vi "Video stream.vi"(0 "VideoMode":u32, 1 "Interface name":T1="cam0", 5 "Video codec":string="Microsoft Video 1", 9 "FPS":u32=30, 11 "Video directory path":path=path "C:/test", 12 "Video name":string="test", 13 "Write video":bool, 14 "Quality":i32=750 max=1000) -> (15 "Error Out":errorcluster)   [LabVIEW 2015]
uses:
  <vilib>/userdefined/High Color/IMAQdx.ctl
  <vilib>/vision/driver/IMAQdx.llb/IMAQdx Camera Control Mode.ctl
  <vilib>/vision/Avi.llb/IMAQ AVI2 Refnum.ctl
  <vilib>/vision/driver/NI_Vision_Acquisition_Software.lvlib
  <resource>/objmgr/imaqdx.rc
panel:
  in  "Stop":bool
  out "Video":T2(plugin-control)
  # "PN 27/11/2014, 27/08/2015 (layout change for web window)"
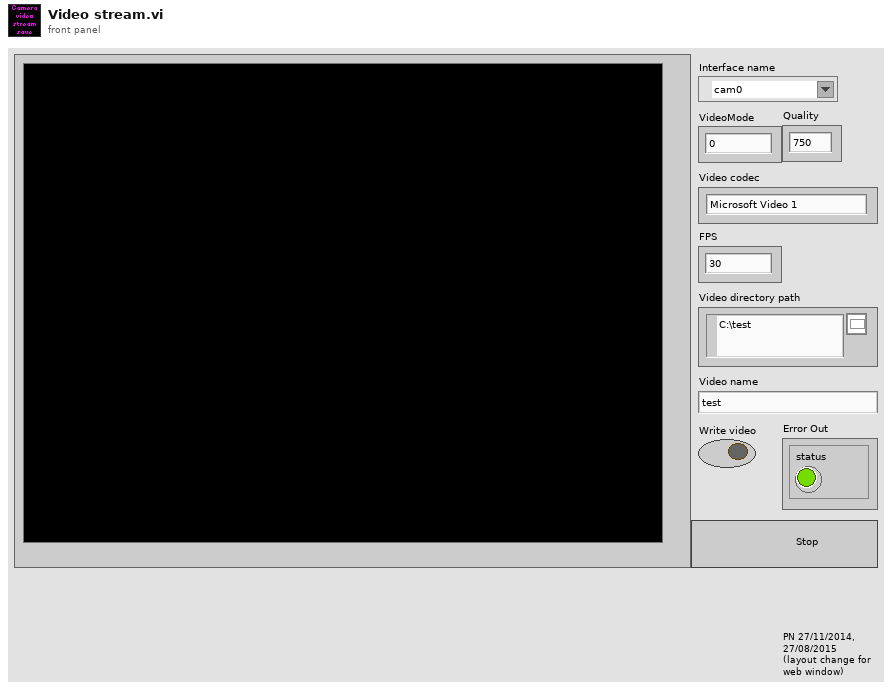
[diagram p1: front panel]
types:
  T1 = typedef "IMAQdx.ctl" = refnum<k21>
  T2 = typedef "IMAQ Image.ctl" = refnum<image>
  T3 = typedef "NI_Vision_Acquisition_Software.lvlib/IMAQdx Camera Control Mode.ctl" = enum32{"Controller", "Listener"}
  T4 = typedef "IMAQ AVI2 Refnum.ctl" = refnum<k20>
  T5 = typedef "Image Type" = u32
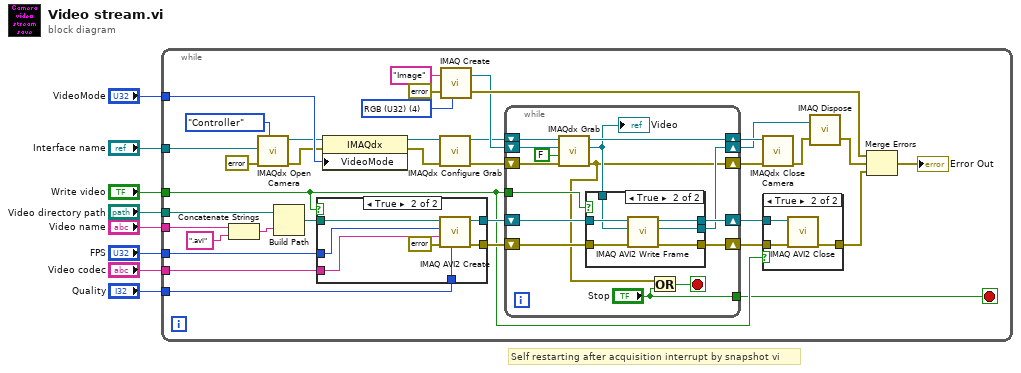
[diagram p0: block diagram]
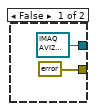
[diagram p2: hidden frame]
diagram:
  # "Self restarting after acquisition interrupt by snapshot vi"
  n1 = while {
    tunnel: "Video directory path" -> [w43]
    tunnel: "Video name" -> [w41]
    tunnel: "Write video" -> [w22]
    tunnel: "VideoMode" -> [w21]
    tunnel: "FPS" -> [w16]
    tunnel: "Interface name" -> [w15]
    tunnel: "Video codec" -> [w13]
    tunnel: "Quality" -> [w9]
    stop <- w12 stop-if-true
    w38 = T5 4 items=["Grayscale (U8)", "Grayscale (I16)", "Grayscale (SGL)", "Complex (CSG)", "RGB (U32)", "HSL (U32)", "RGB (U64)", "Grayscale (U16)"] ("Image Type")
    n2 = Concatenate Strings(w41, ".avi" ("name or relative path")) -> (w40:string)
    n3 = call <vilib>:"IMAQdx Open Camera.vi"("Camera Control Mode"=IMAQdx_Camera_Control_Mode."Controller", "error in"=errorcluster {"status"=FALSE, "code"=0, "source"=""}, "Session In"=w15) -> ("error out"=w18:errorcluster, "Session Out"=w14:T1)  [unwired: 7 in]
    n4 = Build Path(base path=w43, name or relative path=w40) -> (appended path=w32:path)
    n5 = case shown="True" w22 {
      tunnel: w32 -> [_ w53]
      tunnel: [T4 refnum ("AVI Refnum") w52] -> w31
      tunnel: [errorcluster {"status"=FALSE, "code"=0, "source"=""} ("error out") w51] -> w30
      tunnel: w16 -> [_ w50]
      tunnel: w13 -> [_ w49]
      tunnel: w9 -> [_ w47]
      frame False {
      }
      frame True {
        n6 = call "IMAQ AVI2 Create"("Quality"=w47, "error in (no error)"=errorcluster {"status"=FALSE, "code"=0, "source"=""} ("error in"), "Codec"=w49, "Frames Per Second"=w50, "AVI Path"=w53) -> ("error out"=w51:errorcluster, "AVI Refnum"=w52:T4)  [unwired: 5 in]
      }
    }
    n7 = property class="IMAQdx"(reference=w14, error in=w18, "VideoMode"=w21) -> (reference out=w19:T1, error out=w17:errorcluster)
    n8 = call <vilib>:"IMAQdx Configure Grab.vi"("error in"=w17, "Session In"=w19) -> ("error out"=w33:errorcluster, "Session Out"=w20:T1)  [unwired: 8 in]
    n9 = call "IMAQ Create"("Image Name"="Image", "Image Type"=w38, "error in (no error)"=errorcluster {"status"=FALSE, "code"=0, "source"=""} ("error in")) -> ("New Image"=w36:T2, "error out"=w37:errorcluster)  [unwired: 2 in]
    n10 = while {
      shift-right: [w70] -> w35
      shift-left: w20 -> [w72]
      shift-right: [w62] -> w28
      shift-left: w36 -> [w71]
      shift-right: [w60] -> w34
      shift-left: w33 -> [w69]
      tunnel: w22 -> [w67]
      shift-right: [w64] -> w23
      shift-left: w31 -> [w66]
      shift-right: [w61] -> w25
      shift-left: w30 -> [w63]
      tunnel: ["Stop"] -> w12
      stop <- w59 stop-if-true
      n11 = call <vilib>:"IMAQdx Grab.vi"("error in"=w69, "Wait for Next Buffer? (Yes)"=FALSE, "Image In"=w71, "Session In"=w72) -> ("error out"=w60:errorcluster, "Image Out"=w65:T2, "Session Out"=w70:T1)  [unwired: 4 in, 1 out]
      "Video" <- w65
      n12 = case shown="True" w67 {
        tunnel: w66 -> [w75 w81]
        tunnel: w65 -> [w73 w80]
        tunnel: [w75 w79] -> w64
        tunnel: [w74 w78] -> w61
        tunnel: w63 -> [w74 w77]
        tunnel: [w73 w76] -> w62
        frame False {
        }
        frame True {
          n13 = call "IMAQ AVI2 Write Frame"("error in (no error)"=w77, "Image"=w80, "AVI Refnum"=w81) -> ("error out"=w78:errorcluster, "Image Out (duplicate)"=w76:T2, "AVI Refnum (duplicate)"=w79:T4)  [unwired: 6 in]
        }
      }
      n14 = Or(x=w60, y="Stop") -> (x .or. y?=w59:bool)
    }
    n15 = call <vilib>:"IMAQdx Close Camera.vi"("error in"=w34, "Session In"=w35) -> ("error out"=w27:errorcluster)  [unwired: 9 in]
    n16 = case shown="True" w22 {
      tunnel: w25 -> [w54 w57]
      tunnel: [w54 w56] -> w24
      tunnel: w23 -> [_ w55]
      frame False {
      }
      frame True {
        n17 = call "IMAQ AVI2 Close"("error in (no error)"=w57, "AVI Refnum"=w55) -> ("error out"=w56:errorcluster)  [unwired: 9 in]
      }
    }
    n18 = call "IMAQ Dispose"("Image"=w28, "error in (no error)"=w27) -> ("error out"=w26:errorcluster)  [unwired: 4 in]
    n19 = Merge Errors(w37, w26, w24) -> (→"Error Out":errorcluster)
  }
